vi "Handle SmartMotor ASCII strings REVERSE.vi"(3 "error in (no error)":errorcluster, 5 "String in":string) -> (0 "error out":errorcluster, 2 "String out":string)   [LabVIEW 2017]
doc: "Developed by Kevin Thompson\nkevin@thompsonengineering.net\n\nCopyright 2018-2020\nThompson Engineering, LLC"
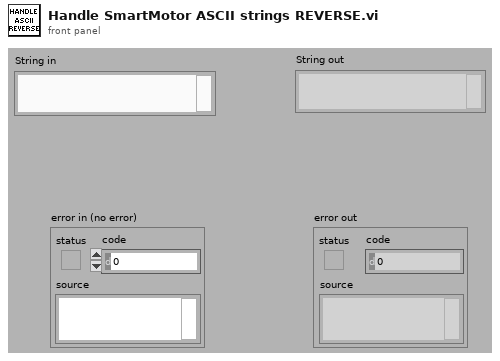
[diagram p1: front panel]
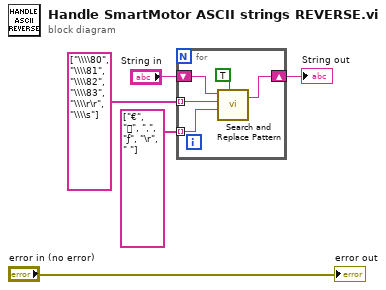
[diagram p0: block diagram]
diagram:
  n1 = for {
    tunnel: string[] ["\\\\80", "\\\\81", "\\\\82", "\\\\83", "\\\\r\r", "\\\\s"] -> [w10] mode=indexing
    shift-right: [w6] -> w1
    shift-left: "String in" -> [w9]
    tunnel: string[] ["€", "", "‚", "ƒ", "\r", " "] -> [w8] mode=indexing
    n2 = call <vilib>:"Search and Replace Pattern.vi"("string"=w9, "regular expression (\"\")"=w10, "replace string (\"\")"=w8, "replace all? (F)"=TRUE) -> ("result string"=w6:string)  [unwired: 1 in, 1 out]
  }
  "String out" <- w1
  "error out" <- "error in (no error)"
